vi "meth.GetPackagePaths.vi"(0 "class.GLue in":refnum<class "class.GLue.lvclass">, 11 "error in":errorcluster, 13 "ms timeout (-1)":i32=-1) -> (4 "class.GLue out":refnum<class "class.GLue.lvclass">, 6 "Lpaths":string, 10 "Cpaths":string, 15 "error out":errorcluster)   [LabVIEW 2014, in "GLue.lvlib" / "class.GLue.lvclass"]
uses:
  class.GLue.lvclass
  class.GLue.lvclass/class.GLue.ctl
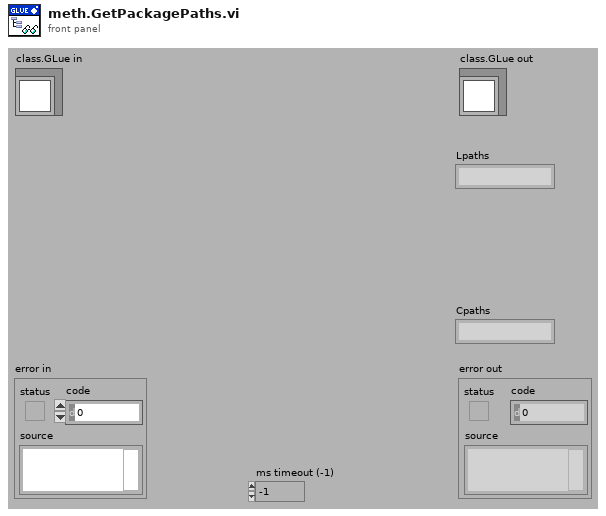
[diagram p1: front panel]
types:
  T1 = typedef "Semaphore RefNum" = refnum<k1>
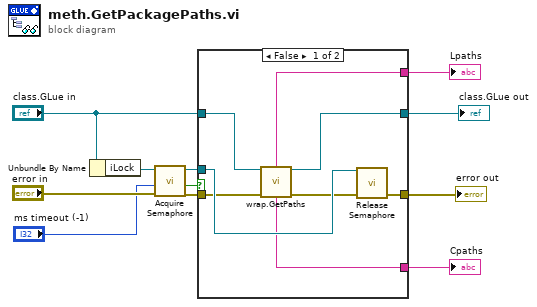
[diagram p0: block diagram]
diagram:
  n1 = Unbundle By Name("class.GLue in") -> ("iLock"=w11:T1)
  n2 = call <vilib>:"Acquire Semaphore.vi"("error in (no error)"="error in", "ms timeout (-1)"="ms timeout (-1)", "semaphore"=w11) -> ("error out"=w10:errorcluster, "timed out"=w9:bool, "semaphore out"=w8:T1)  [unwired: 2 in]
  n3 = case shown="False" w9 {
    tunnel: [w19 w20] -> w3
    tunnel: [w16 w21] -> w4
    tunnel: "class.GLue in" -> [w17 w21]
    tunnel: w10 -> [w15 w20]
    tunnel: w8 -> [w18 _]
    tunnel: [w13 _] -> w2
    tunnel: [w12 _] -> w1
    frame False {
      n4 = call "wrap.GetPaths.vi"("class.GLue in"=w17, "error in (no error)"=w15) -> ("Lpaths"=w13:string, "class.GLue out"=w16:refnum<class "class.GLue.lvclass">, "Cpaths"=w12:string, "error out"=w14:errorcluster)  [unwired: 10 in]
      n5 = call <vilib>:"Release Semaphore.vi"("error in (no error)"=w14, "semaphore"=w18) -> ("error out"=w19:errorcluster)  [unwired: 4 in, 1 out]
    }
    frame True {
    }
  }
  "error out" <- w3
  "class.GLue out" <- w4
  "Lpaths" <- w2
  "Cpaths" <- w1
